vi "Fetch (Measurement).vi"(7 "Measurement (0:Frequency)":i32(ring) items=["Frequency", "Frequency Ratio", "Period", "Totalize", "Phase", "Edge Rise Time", "Edge Fall Time", "Positive Pulse Width", "Negative Pulse Width", "Duty Cycle", "Time Interval", "Volt Maximum", "Volt Minimum"], 8 "error in (no error)":errorcluster, 10 "Totalize Arm Type (0:Time/External)":i32(ring) items=["Time/External", "Auto"], 11 "VISA resource name":refnum<visa-resource-name>) -> (0 "error out":errorcluster, 2 "Result":dbl format="%#.10g", 3 "VISA resource name out":refnum<visa-resource-name>)   [LabVIEW 2013, in "Counter.lvlib" / "PICOTEST U62XXA series.lvlib"]
doc: "Queries and retrieves measurement results.\n\n<B>Note:</B>\n\nIf no valid result exists, Not a Number 9.91E37 is returned."
uses:
  PICOTEST U62XXA series.lvlib
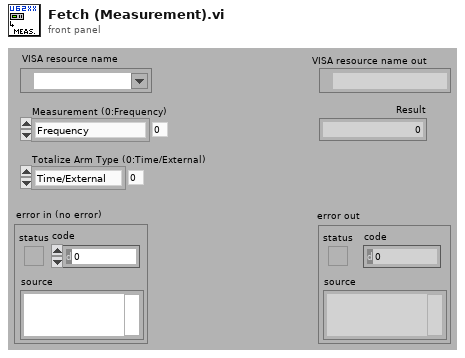
[diagram p1: front panel]
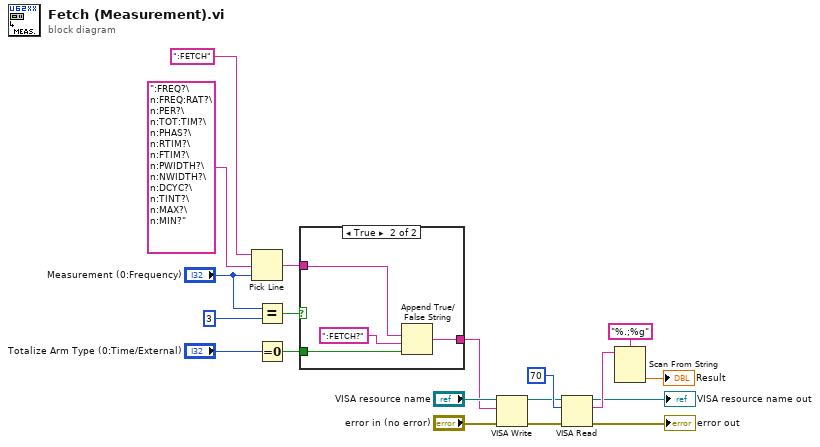
[diagram p0: block diagram]
diagram:
  n1 = Pick Line(string ("")=":FETCH", multi-line string=":FREQ?\n:FREQ:RAT?\n:PER?\n:TOT:TIM?\n:PHAS?\n:RTIM?\n:FTIM?\n:PWIDTH?\n:NWIDTH?\n:DCYC?\n:TINT?\n:MAX?\n:MIN?", line index="Measurement (0:Frequency)") -> (output string=w6:string)
  n2 = Equal?(x="Measurement (0:Frequency)", y=3 ("x")) -> (x = y?=w4:bool)
  n3 = Equal To 0?(x="Totalize Arm Type (0:Time/External)") -> (x = 0?=w3:bool)
  n4 = case shown="True" w4 {
    tunnel: [w20 w24] -> w7
    tunnel: w6 -> [w20 w22]
    tunnel: w3 -> [_ w23]
    frame False {
    }
    frame True {
      n5 = Append True/False String(1:w23, 2:":FETCH?", 3:w22) -> (0:w24:string)  [unwired: 1 in]
    }
  }
  n6 = VISA Write(VISA resource name="VISA resource name", write buffer=w7, error in (no error)="error in (no error)") -> (VISA resource name out=w9:refnum<visa-resource-name>, error out=w10:errorcluster)  [unwired: 1 out]
  n7 = VISA Read(VISA resource name=w9, byte count=u32 70, error in (no error)=w10) -> (VISA resource name out=→"VISA resource name out":refnum<visa-resource-name>, read buffer=w17:string, error out=→"error out":errorcluster)  [unwired: 1 out]
  n8 = Scan From String(format string="%.;%g", input string=w17) -> (output 1=→"Result":dbl)  [unwired: 3 in, 3 out]
